vi "API_Get Cursor Position.vi"() -> ()   [LabVIEW 2011, in "API.lvlib"]
doc: "This VI returns the mouse position in screen coordinates."
uses:
  API.lvlib
  user32.dll
panel:
  out "Cursor Pos":cluster{"x":i16, "y":i16}
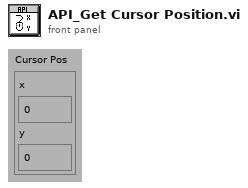
[diagram p1: front panel]
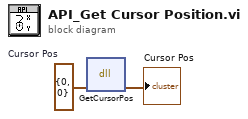
[diagram p0: block diagram]
diagram:
  w2 = cluster{"x":i32, "y":i32} {"x"=0, "y"=0}  # Cursor Pos
  n1 = dll-call lib="user32.dll" fn="GetCursorPos"(w2) -> (→"Cursor Pos":cluster{"x":i32, "y":i32})  [unwired: 4 in, 2 out]
